vi "Global.vi"() -> ()   [LabVIEW 2016]
uses:
  <vilib>/vision/Image Controls.llb/IMAQ Image.ctl
  ctl/force_sensor_data.ctl
panel:
  out "Balance_xy_p":cluster{dbl, dbl}[](array[cluster])
  in  "force_low_level":dbl
  in  "save drive":string="c:\\"
  in  "cDAQ_config":T1
  out "Force Sensor data":T2
  in  "Simulation config":T3 {"simulation speed" scale=0.0..1000.0}
  in  "simulation file path":path
  in  "simulation":bool
  out "force_cal":dbl
  in  "Temp offset":dbl=37.0
  out "minmin df":dbl
  in  "Strain 4x":bool
  out "Image Out":T4
  out "ROI":T5
  in  "stop":bool
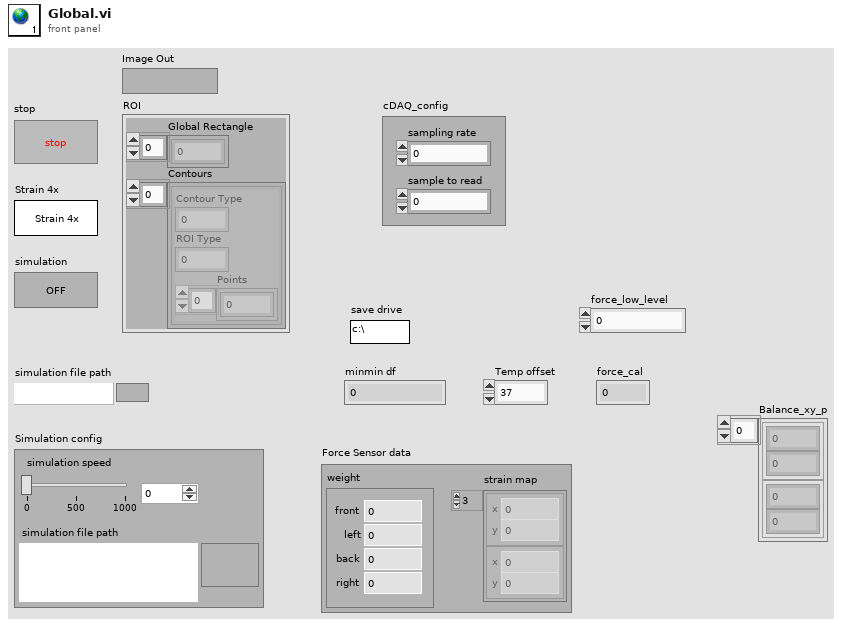
[diagram p1: front panel]
types:
  T1 = cluster{"sampling rate":dbl, "sample to read":dbl}
  T2 = typedef "force_sensor_data.ctl" = cluster{"weight":cluster{"front":dbl, "left":dbl, "back":dbl, "right":dbl}, "strain map":cluster{"x":dbl, "y":dbl}[]}
  T3 = cluster{"simulation file path":path, "simulation speed":u32}
  T4 = typedef "IMAQ Image.ctl" = refnum<image>
  T5 = cluster{"Global Rectangle":i32[], "Contours":cluster{"Contour Type":u32, "ROI Type":u32, "Points":i32[]}[]}
diagram:
